vi "Gyro Straightening.vi"(8 "Gyro Setpoint":dbl, 9 "Right Drive Power":dbl, 10 "Left Drive Power":dbl, 11 "Gyro Angle":dbl) -> (1 "Right Drive":dbl, 2 "Left Drive":dbl)   [LabVIEW 2011]
panel:
  in  "Lower Limit":dbl=1.0
  in  "Upper Limit":dbl=1.0
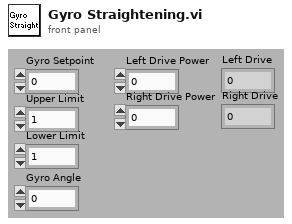
[diagram p1: front panel]
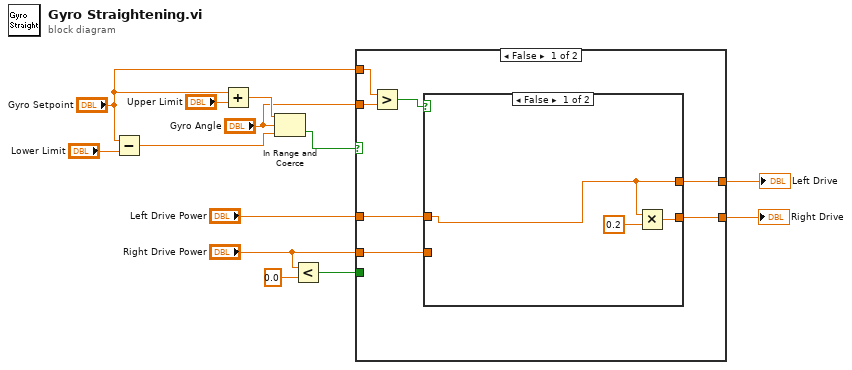
[diagram p0: block diagram]
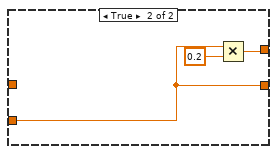
[diagram p2: hidden frame]
diagram:
  n1 = Subtract(x="Gyro Setpoint", y="Lower Limit") -> (x-y=w7:dbl)
  n2 = Add(x="Gyro Setpoint", y="Upper Limit") -> (x+y=w9:dbl)
  n3 = In Range and Coerce(upper limit=w9, x="Gyro Angle", lower limit=w7) -> (In Range?=w13:bool)  [unwired: 1 out]
  n4 = Less?(x="Right Drive Power", y=0.0) -> (x < y?=w1:bool)
  n5 = case shown="False" w13 {
    tunnel: "Gyro Setpoint" -> [w19 _]
    tunnel: "Gyro Angle" -> [w18 _]
    tunnel: "Left Drive Power" -> [w17 w28]
    tunnel: "Right Drive Power" -> [w16 w27]
    tunnel: [w15 w28] -> w11
    tunnel: [w14 w27] -> w10
    tunnel: w1 -> [_ _]
    frame False {
      n6 = Greater?(x=w19, y=w18) -> (0:w20:bool)
      n7 = case shown="False" w20 {
        tunnel: w17 -> [w22 _]
        tunnel: w16 -> [_ w25]
        tunnel: [w22 w26] -> w15
        tunnel: [w23 w25] -> w14
        frame False {
          n8 = Multiply(x=w22, y=0.2) -> (x*y=w23:dbl)
        }
        frame True {
          n9 = Multiply(x=w25, y=0.2) -> (x*y=w26:dbl)
        }
      }
    }
    frame True {
    }
  }
  "Left Drive" <- w11
  "Right Drive" <- w10
